vi "main.vi"() -> ()   [LabVIEW 2022 SP3]
uses:
  <vilib>/Instr/_visa.llb/VISA Configure Serial Port (Instr).vi
  C:/Program Files/National Instruments/LabVIEW 2022/examples/Instrument IO/Serial/support/Serial - ASCII Characters.ctl
  C:/Program Files/National Instruments/LabVIEW 2022/examples/Instrument IO/Serial/support/Serial - XON-XOFF Characters.ctl
  C:/Program Files/National Instruments/LabVIEW 2022/examples/Instrument IO/Serial/support/Serial - Settings.ctl
panel:
  in  "Termination Character":u8=10 format="%.0x"
  in  "End Write on Termination Character?":bool=TRUE
  in  "VISA resource name":refnum<visa-resource-name>="COM1"
  in  "End Read on Termination Character?":bool=TRUE
  out "Response":string
  in  "Read Count":u32=1000
  in  "Command":string="*IDN?"
  in  "Read":bool
  in  "Write":bool
  out "Waveform Chart":dbl(graph)
  in  "Simullation parameters":T1={"static gain"=2.5, "lag (s)"=2.5, "deadtime (s)"=0.001, "load"=0.0, "deadband"=0.0, "sensor noise"=0.0, "initial PV"=0.2, "plant noise"=0.0} {"plant noise" format="%.2f"; "initial PV" format="%.2f"; "sensor noise" format="%.2f"; "lag (s)" format="%.2f"; "deadtime (s)" format="%.2f"; "deadband" format="%.1f"; "load" format="%.2f"; "static gain" format="%.2f"}
  in  "reinitialize? (F)":bool
  in  "dt (s)":dbl=0.3 format="%.3f"
  in  "output saturation range":cluster{"output high":dbl, "output low":dbl}={"output high"=inf, "output low"=-inf}
  in  "stop":bool
  in  "Pump flow":dbl(slide) scale=0.0..10.0
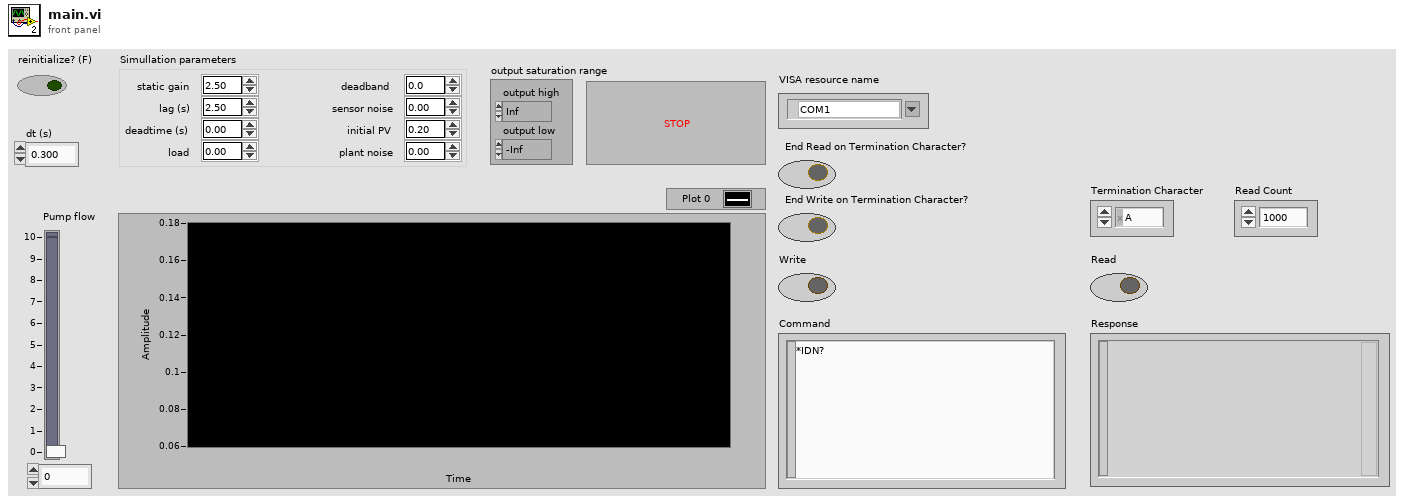
[diagram p1: front panel]
types:
  T1 = cluster{"static gain":dbl, "lag (s)":dbl, "deadtime (s)":dbl, "load":dbl, "deadband":dbl, "sensor noise":dbl, "initial PV":dbl, "plant noise":dbl}
  T2 = typedef "Serial - Settings.ctl" = cluster{"baud rate":u32, "data bits":u16, "parity":enum16{"None", "Odd", "Even", "Mark", "Space"}, "stop bits":u16, "flow control":u16}
  T3 = typedef "Serial - XON-XOFF Characters.ctl" = cluster{"XON":T4, "XOFF":T4}
  T4 = typedef "Serial - ASCII Characters.ctl" = enum16{"NUL", "SOH", "STX", "ETX", "EOT", "ENQ", "ACK", "BEL", "BS", "HT", "LF", "VT", "FF", "CR", "SO", "SI", "DLE", "DC1", "DC2", "DC3", "DC4", "NAK", "SYN", "ETB", "CAN", "EM", "SUB", "ESC", "FS", "GS", "RS", "US", "SP", "!", "\"", "#", "$", "%", "&", "'", "(", ")", "*", "+", ",", "- (-)", ".", "/", "0", "1", "2", "3", "4", "5", "6", "7", "8", "9", ":", ";", "<", "=", ">", "?", "@", "A", "B", "C", "D", "E", "F", "G", "H", "I", "J", "K", "L", "M", "N", "O", "P", "Q", "R", "S", "T", "U", "V", "W", "X", "Y", "Z", "[", "\\", "]", "^", "_", "`", "a", "b", "c", "d", "e", "f", "g", "h", "i", "j", "k", "l", "m", "n", "o", "p", "q", "r", "s", "t", "u", "v", "w", "x", "y", "z", "{", "|", "}", "~"}
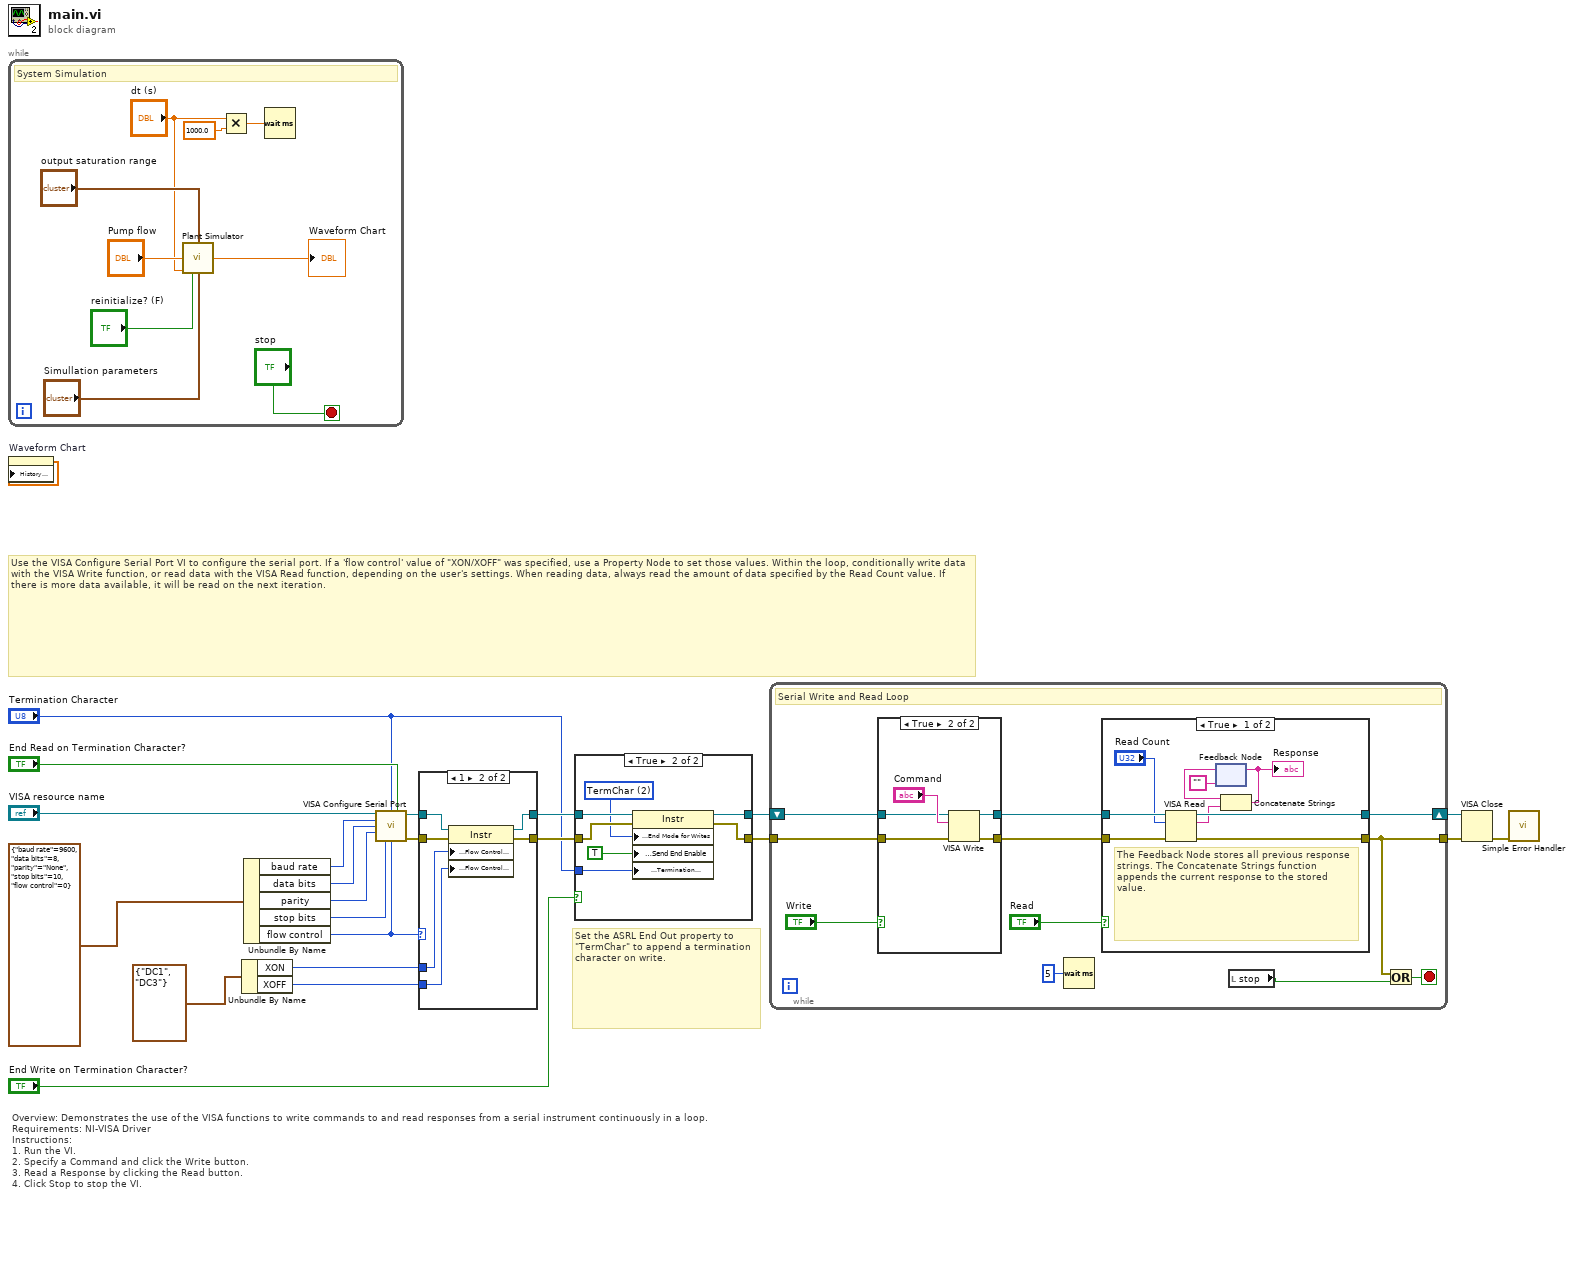
[diagram p0: block diagram]
diagram:
  # "Set the ASRL End Out property to \"TermChar\" to append a termination character on write."
  # "Use the VISA Configure Serial Port VI to configure the serial port. If a 'flow control' value of \"XON/XOFF\" was specified, use a Property Node to set those values. Within the loop, conditionally write data with the VISA Write function, or read data with the VISA Read function, depending on the user's settings. When reading data, always read the amount of data specified by the Read Count value. If there is more data available, it will be read on the next iteration."
  # "Overview: Demonstrates the use of the VISA functions to write commands to and read responses from a serial instrument continuously in a loop.\nRequirements: NI-VISA Driver\nInstructions:\n1. Run the VI.\n2. Specify a Command and click the Write button.\n3. Read a Response by clicking the Read button.\n4. Click Stop to stop the VI."
  n1 = while {
    stop <- "stop" stop-if-true
    # "System Simulation"
    n2 = call "Plant Simulator.vi"("output saturation range"="output saturation range", "Plant Input"="Pump flow", "dt (s)"="dt (s)", "reinitialize? (F)"="reinitialize? (F)", "Simullation parameters"="Simullation parameters") -> ("Plant Output"=→"Waveform Chart":dbl)  [unwired: 10 in]
    n3 = Multiply(x="dt (s)", y=1000.0) -> (x*y=w24:dbl)
    n4 = Wait (ms)(milliseconds to wait=w24) -> ()  [unwired: 1 out]
  }
  n5 = property on="Waveform Chart" class="WFChart (strict)"("History Data"=dbl[] []) -> ()  [unwired: 2 in, 2 out]
  n6 = Unbundle By Name(T3 {"XON"=enum."DC1", "XOFF"=enum."DC3"} ("XON/XOFF Characters")) -> ("XON"=w8:T4, "XOFF"=w7:T4)
  n7 = Unbundle By Name(T2 {"baud rate"=9600, "data bits"=8, "parity"=enum."None", "stop bits"=10, "flow control"=0} ("Serial Settings")) -> ("baud rate"=w15:u32, "data bits"=w16:u16, "parity"=w17:enum16{"None", "Odd", "Even", "Mark", "Space"}, "stop bits"=w18:u16, "flow control"=w9:u16)
  n8 = call-poly "VISA Configure Serial Port"("VISA resource name"="VISA resource name", "termination char\n(0xA = '\\n' = LF)"="Termination Character", "Enable Termination\nChar (T)"="End Read on Termination Character?", "baud rate (9600)"=w15, "data bits (8)"=w16, "parity (0:none)"=w17, "stop bits (10: 1 bit)"=w18, "flow control (0:none)"=w9) -> ("VISA resource name out"=w19:refnum<visa-resource-name>, "error out"=w20:errorcluster)  [unwired: 2 in, 4 out]
  n9 = case shown="1" w9 {
    tunnel: [w33 w40] -> w6
    tunnel: [w34 w39] -> w4
    tunnel: w20 -> [w33 w38]
    tunnel: w19 -> [w34 w37]
    tunnel: w8 -> [_ w36]
    tunnel: w7 -> [_ w35]
    frame Default {
    }
    frame 1 {
      n10 = property class="Instr"(reference=w37, error in=w38, "Serial Settings:Flow Control XON Character"=w36, "Serial Settings:Flow Control XOFF Character"=w35) -> (reference out=w39:refnum<visa-resource-name>, error out=w40:errorcluster)
    }
  }
  n11 = case shown="True" "End Write on Termination Character?" {
    tunnel: w4 -> [w41 w49]
    tunnel: w6 -> [w42 w48]
    tunnel: [w41 w47] -> w3
    tunnel: [w42 w46] -> w5
    tunnel: "Termination Character" -> [_ w44]
    frame False {
    }
    frame True {
      w45 = u16 2 items=["None", "LastBit", "TermChar", "Break"] ("Serial Settings:Serial End Mode for Writes")
      n12 = property class="Instr"(reference=w49, error in=w48, "Serial Settings:End Mode for Writes"=w45, "Message Based Settings:Send End Enable"=TRUE, "Message Based Settings:Termination Character"=w44) -> (reference out=w47:refnum<visa-resource-name>, error out=w46:errorcluster)
    }
  }
  n13 = while {
    shift-right: [w60] -> w10
    shift-left: w3 -> [w59]
    tunnel: w5 -> [w58]
    tunnel: [w52] -> w11
    stop <- w53 stop-if-true
    # "Serial Write and Read Loop"
    n14 = case shown="True" "Write" {
      tunnel: w59 -> [w62 w66]
      tunnel: w58 -> [w61 w65]
      tunnel: [w62 w64] -> w57
      tunnel: [w61 w63] -> w56
      frame False {
      }
      frame True {
        n15 = VISA Write(VISA resource name=w66, write buffer="Command", error in (no error)=w65) -> (VISA resource name out=w64:refnum<visa-resource-name>, error out=w63:errorcluster)  [unwired: 1 out]
      }
    }
    n16 = Wait (ms)(milliseconds to wait=u32 5) -> ()  [unwired: 1 out]
    n17 = case shown="True" "Read" {
      tunnel: [w74 w78] -> w60
      tunnel: w57 -> [w76 w78]
      tunnel: [w72 w77] -> w52
      tunnel: w56 -> [w75 w77]
      frame True {
        # "The Feedback Node stores all previous response strings. The Concatenate Strings function appends the current response to the stored value."
        n18 = VISA Read(VISA resource name=w76, byte count="Read Count", error in (no error)=w75) -> (VISA resource name out=w74:refnum<visa-resource-name>, read buffer=w71:string, error out=w72:errorcluster)  [unwired: 1 out]
        n19 = feedback #1("") -> (w70:string)
        n20 = Concatenate Strings(w70, w71) -> (w69:string)
        "Response" <- w69
        n21 = feedback-in #1(w69) -> ()
      }
      frame False {
      }
    }
    n22 = local read "stop"() -> (w50:bool)
    n23 = Or(x=w52, y=w50) -> (x .or. y?=w53:bool)
  }
  n24 = VISA Close(VISA resource name=w10, error in (no error)=w11) -> (error out=w12:errorcluster)
  n25 = call <vilib>:"Simple Error Handler.vi"("error in (no error)"=w12) -> ()  [unwired: 1 in, 8 out]
